vi "UnLoad.vi"(8 "error in (no error)":errorcluster) -> (0 "error out":errorcluster)   [LabVIEW 2017, in "WebServiceImporter.lvlib" / "Main Panel.lvlib" / "Preview.lvlib"]
uses:
  <vilib>/Platform/WebService/Main Panel/Pages/Preview/Preview.lvlib
  <vilib>/Platform/WebService/Main Panel/Pages/Preview/Events/Events.lvlib
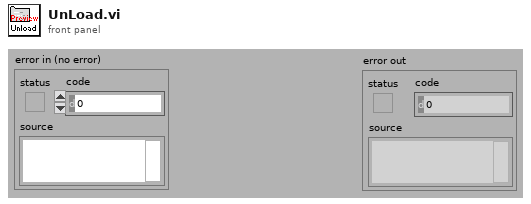
[diagram p1: front panel]
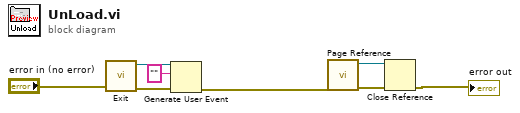
[diagram p0: block diagram]
diagram:
  n1 = call <vilib>:"Exit.vi"("error in (no error)"="error in (no error)") -> ("error out"=w2:errorcluster, "user event (out)"=w4:refnum<user-event>)  [unwired: 9 in]
  n2 = Generate User Event(user event=w4, event data cluster="" ("event data"), error in=w2) -> (error out=w1:errorcluster)  [unwired: 1 in, 1 out]
  n3 = call <vilib>:"Page Reference.vi"("error in (no error)"=w1) -> ("error out"=w5:errorcluster, "VI Refnum (out)"=w6:refnum<vi>)  [unwired: 9 in]
  n4 = Close Reference(reference=w6, error in (no error)=w5) -> (error out=→"error out":errorcluster)
